vi "Elf2DataRecord.vi"(8 "Error In":errorcluster, 11 "Elf file":path) -> (0 "error out":errorcluster, 3 "DataRecord":T1 {"Address" format="%.0x"; "Data" format="%.0x"})   [LabVIEW 2015]
uses:
  DataControl.ctl
panel:
  out "Parsed SREC":string
  out "NumRecords":i32
  out "filename without extension":string
  # "C:\\Users\\8135cont24\\Desktop\\Demo\\aPAN2\\APAN\\mb-DMAboot\\mb-DMAboot\\xsdk_worspace\\helloworld1\\Debug\\helloworld1.elf"
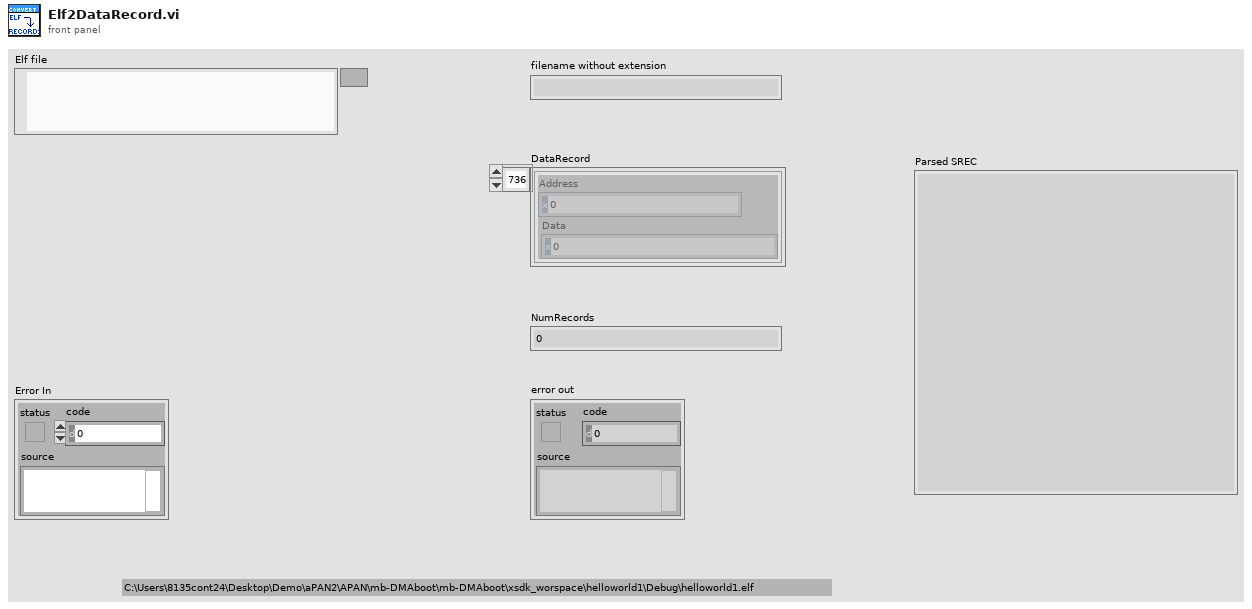
[diagram p1: front panel]
types:
  T1 = typedef "DataControl.ctl" = cluster{"Address":u32, "Data":u32}[]
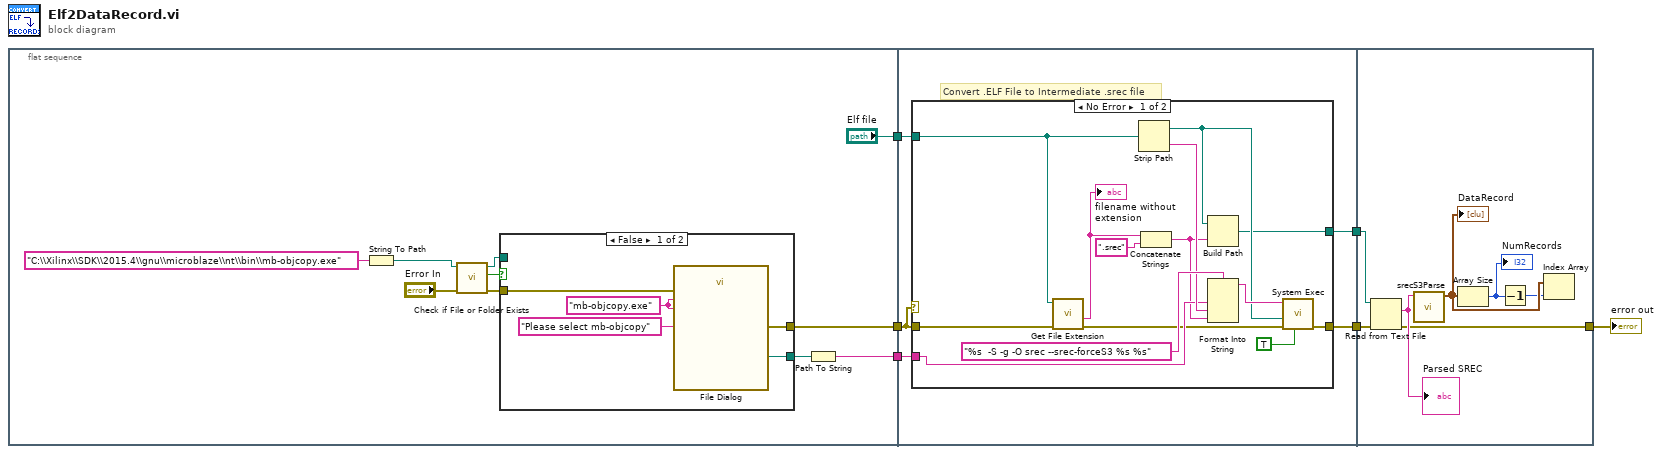
[diagram p0: block diagram]
diagram:
  n1 = flat-sequence {
    tunnel: ["Elf file"] -> w6
    tunnel: [w10] -> w5
    tunnel: [w7] -> w3
    tunnel: w6 -> [w27]
    tunnel: w5 -> [w28]
    tunnel: [w26] -> w4
    tunnel: w3 -> [w24]
    tunnel: [w25] -> w2
    tunnel: w4 -> [w51]
    tunnel: w2 -> [w46]
    tunnel: [w45] -> w1
    frame #0 {
      n2 = String To Path(string="C:\\Xilinx\\SDK\\2015.4\\gnu\\microblaze\\nt\\bin\\mb-objcopy.exe") -> (path=w15:path)
      n3 = call <vilib>:"Check if File or Folder Exists.vi"("error in (no error)"="Error In", "path"=w15) -> ("error out"=w8:errorcluster, "file or folder exists?"=w14:bool, "dup path"=w13:path)  [unwired: 7 in]
      n4 = case shown="False" w14 {
        tunnel: w13 -> [_ w23]
        tunnel: [w21 w23] -> w11
        tunnel: w8 -> [w18 w22]
        tunnel: [w17 w22] -> w7
        frame False {
          w19 = "mb-objcopy.exe" ("pattern label")
          n5 = call "File Dialog"("prompt"="Please select mb-objcopy", "error in"=w18, "pattern (all files)"=w19, "pattern label"=w19) -> ("selected path"=w21:path, "error out"=w17:errorcluster)  [unwired: 8 in, 2 out]
        }
        frame True {
        }
      }
      n6 = Path To String(path=w11) -> (string=w10:string)
    }
    frame #1 {
      # "Convert .ELF File to Intermediate .srec file"
      n7 = case shown="No Error" w24 {
        tunnel: w28 -> [w40 _]
        tunnel: w27 -> [w39 w44]
        tunnel: [w32 w44] -> w26
        tunnel: w24 -> [w31 w43]
        tunnel: [w29 w43] -> w25
        frame No Error {
          n8 = call <vilib>:"Get File Extension.vi"("error in (no error)"=w31, "file"=w39) -> ("error out"=w30:errorcluster, "filename without extension"=w38:string)  [unwired: 5 in, 3 out]
          "filename without extension" <- w38
          n9 = Strip Path(path=w39) -> (stripped path=w33:path, name=w41:string)
          n10 = Concatenate Strings(w38, ".srec" ("string")) -> (w34:string)
          n11 = Build Path(base path=w33, name or relative path=w34) -> (appended path=w32:path)
          n12 = Format Into String(format string="%s  -S -g -O srec --srec-forceS3 %s %s", w40, w41, w34) -> (resulting string=w35:string)  [unwired: 2 in, 1 out]
          n13 = call <vilib>:"System Exec.vi"("run minimized? (F)"=TRUE, "error in (no error)"=w30, "working directory"=w33, "command line"=w35) -> ("error out"=w29:errorcluster)  [unwired: 4 in, 3 out]
        }
        frame Error {
        }
      }
    }
    frame #2 {
      n14 = Read from Text File(file (use dialog)=w51, error in=w46) -> (text=w50:string, error out=w45:errorcluster)  [unwired: 2 in, 2 out]
      "Parsed SREC" <- w50
      n15 = call "srecS3Parse.vi"("SrecS3"=w50) -> ("DataRecord"=w49:cluster{"Address":u32, "Data":u32}[])  [unwired: 10 in]
      "DataRecord" <- w49
      n16 = Array Size(array=w49) -> (size(s)=w48:i32)
      "NumRecords" <- w48
      n17 = Decrement(x=w48) -> (x-1=w47:i32)
      n18 = Index Array(array=w49, index=w47) -> ()  [unwired: 1 out]
    }
  }
  "error out" <- w1
